vi "Create_Command.vi"(8 "error in":errorcluster, 9 "On/OFF":bool, 10 "Select":bool, 11 "Intensity":u8 max=100 step=1) -> (0 "error out":errorcluster, 3 "Command":string)   [LabVIEW 2025]
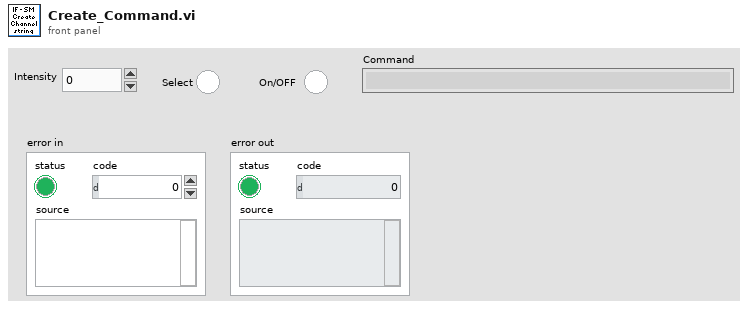
[diagram p1: front panel]
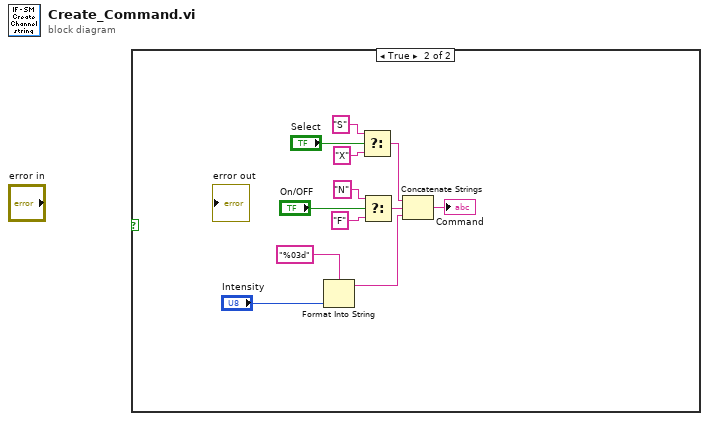
[diagram p0: block diagram]
diagram:
  n1 = case shown="True" {
    selector: _ -> [_ _]
    frame False {
    }
    frame True {
      n2 = Format Into String(format string="%03d", "Intensity") -> (resulting string=w1:string)  [unwired: 2 in, 1 out]
      n3 = Select(t="S" ("string"), s="Select", f="X" ("string")) -> (s? t:f=w12:string)
      n4 = Select(t="N" ("string"), s="On/OFF", f="F" ("string")) -> (s? t:f=w5:string)
      n5 = Concatenate Strings(w12, w5, w1) -> (→"Command":string)
    }
  }
